vi "I32 to Hex(4 Bytes)(SubVI).vi"(8 "error in (no error)":errorcluster, 11 "I32":i32) -> (0 "BYTE 3":string, 1 "BYTE 2":string, 2 "BYTE1":string, 3 "BYTE 0":string, 4 "error out":errorcluster)   [LabVIEW 2014, in "CAP-USB.lvlib"]
doc: "Separa el numero de 32 bits de la entrada\nen sus 4 componentes de 8 bits"
uses:
  CAP-USB.lvlib
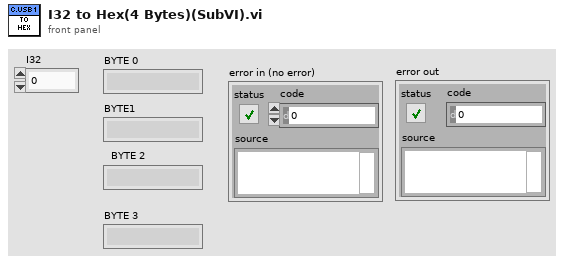
[diagram p1: front panel]
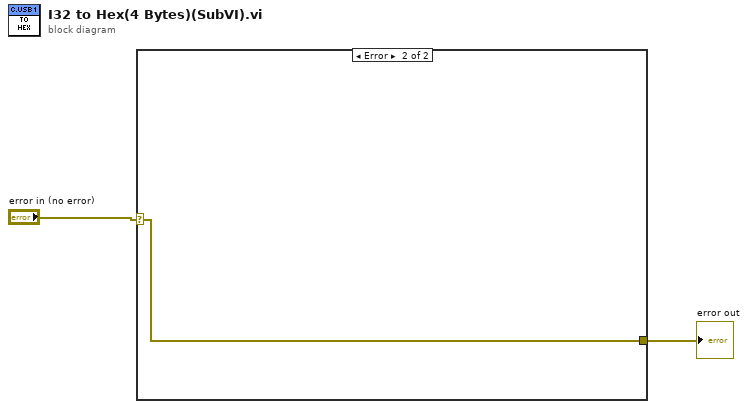
[diagram p0: block diagram]
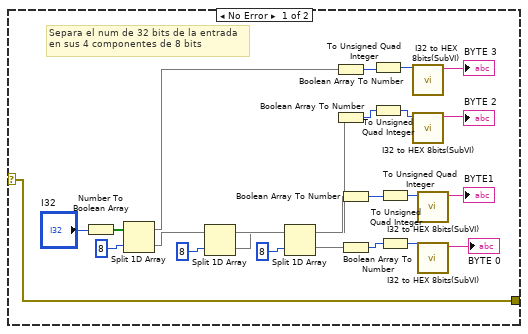
[diagram p2: hidden frame]
diagram:
  n1 = case shown="Error" "error in (no error)" {
    selector: "error in (no error)" -> [w3 w27]
    tunnel: [w3 w27] -> w1
    frame No Error {
      # "Separa el num de 32 bits de la entrada\nen sus 4 componentes de 8 bits"
      n2 = Number To Boolean Array(number="I32") -> (Boolean array=w13:bool[])
      n3 = Split 1D Array(array=w13, index=8) -> (first subarray=w18:bool[], second subarray=w15:bool[])
      n4 = Split 1D Array(array=w15, index=8) -> (first subarray=w19:bool[], second subarray=w17:bool[])
      n5 = Split 1D Array(array=w17, index=8) -> (first subarray=w20:bool[], second subarray=w21:bool[])
      n6 = Boolean Array To Number(Boolean array=w18) -> (number=w11:u32)
      n7 = Boolean Array To Number(Boolean array=w19) -> (number=w8:u32)
      n8 = Boolean Array To Number(Boolean array=w20) -> (number=w6:u32)
      n9 = Boolean Array To Number(Boolean array=w21) -> (number=w4:u32)
      n10 = To Unsigned Quad Integer(1:w11) -> (0:w10:u64)
      n11 = To Unsigned Quad Integer(1:w8) -> (0:w9:u64)
      n12 = To Unsigned Quad Integer(1:w6) -> (0:w7:u64)
      n13 = To Unsigned Quad Integer(1:w4) -> (0:w5:u64)
      n14 = call "I32 to HEX 8bits(SubVI).vi"("IN U64"=w10) -> ("OUT HEX 8BITS"=→"BYTE 3":string)  [unwired: 10 in]
      n15 = call "I32 to HEX 8bits(SubVI).vi"("IN U64"=w9) -> ("OUT HEX 8BITS"=→"BYTE 2":string)  [unwired: 10 in]
      n16 = call "I32 to HEX 8bits(SubVI).vi"("IN U64"=w7) -> ("OUT HEX 8BITS"=→"BYTE1":string)  [unwired: 10 in]
      n17 = call "I32 to HEX 8bits(SubVI).vi"("IN U64"=w5) -> ("OUT HEX 8BITS"=→"BYTE 0":string)  [unwired: 10 in]
    }
    frame Error {
    }
  }
  "error out" <- w1
